vi "Draw Circle.vi"(1 "scale":dbl, 2 "y":dbl, 3 "x":dbl) -> (0 "output cluster":cluster{dbl[], dbl[]})   [LabVIEW 2011]
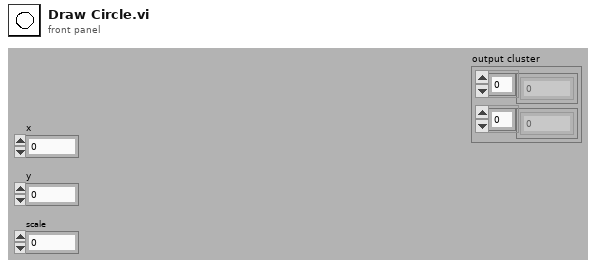
[diagram p1: front panel]
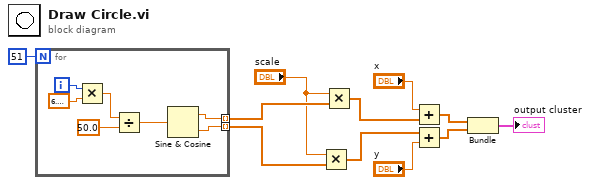
[diagram p0: block diagram]
diagram:
  n1 = for {
    N: 51 -> [_]
    tunnel: [w13] -> w6 mode=indexing
    tunnel: [w12] -> w5 mode=indexing
    i -> [w18]
    n2 = Multiply(x=w18, y=6.283185307179586) -> (x*y=w16:dbl)
    n3 = Divide(x=w16, y=50.0) -> (x/y=w14:dbl)
    n4 = Sine & Cosine(0:w14) -> (1:w13:dbl, 2:w12:dbl)
  }
  n5 = Multiply(x="scale", y=w5) -> (x*y=w3:dbl[])
  n6 = Multiply(x="scale", y=w6) -> (x*y=w2:dbl[])
  n7 = Add(x="x", y=w2) -> (x+y=w9:dbl[])
  n8 = Add(x=w3, y="y") -> (x+y=w10:dbl[])
  n9 = Bundle(w9, w10) -> (→"output cluster":cluster{dbl[], dbl[]})  [unwired: 1 in]
